vi "Running State Logic.vi"(8 "error in (no error)":errorcluster, 11 "CIFCorePlugin in":refnum<class "CIFCorePlugin.lvclass">) -> (0 "error out":errorcluster, 2 "Running State Logic":T1, 3 "CIFCorePlugin out":refnum<class "CIFCorePlugin.lvclass">)   [LabVIEW 2021, in "CIFCorePlugin.lvclass"]
uses:
  CIFCorePlugin.lvclass
  Typedef/Running State Logic.ctl
  CIFCorePlugin.lvclass/CIFCorePlugin.ctl
  Common/Typedef/Plugin State.ctl
  Common/CIFCoreCommon.lvlib
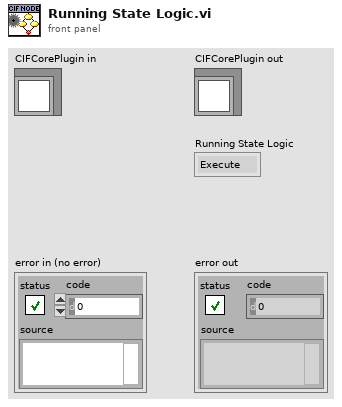
[diagram p1: front panel]
types:
  T1 = typedef "CIFCorePlugin.lvclass/Running State Logic.ctl" = enum16{"Execute", "Housekeep", "Cleanup", "Error", "Destroy"}
  T2 = typedef "CIFCorePlugin.lvclass/Energized States.ctl" = enum16{"Listen", "Prepare", "Execute", "Housekeep", "Cleanup", "Destroy"}
  T3 = typedef "CIFCoreCommon.lvlib/Plugin State.ctl" = enum32{"Null", "Creating", "Listening", "Running", "CleaningUp", "Destroying"}
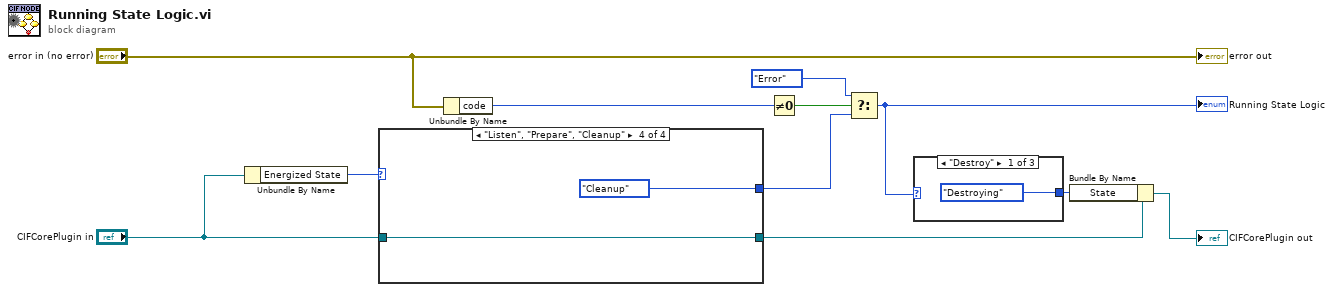
[diagram p0: block diagram]
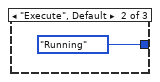
[diagram p2: hidden frame]
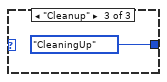
[diagram p3: hidden frame]
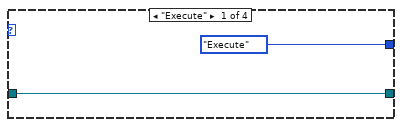
[diagram p4: hidden frame]
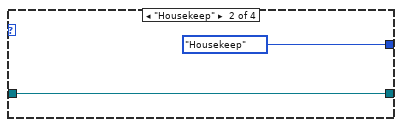
[diagram p5: hidden frame]
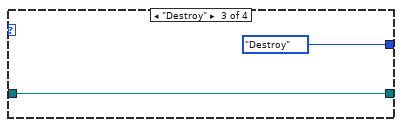
[diagram p6: hidden frame]
diagram:
  n1 = Unbundle By Name("CIFCorePlugin in") -> ("Energized State"=w8:T2)
  n2 = case shown="\"Listen\", \"Prepare\", \"Cleanup\"" w8 {
    tunnel: [Running_State_Logic."Execute" ("Execute State Logic") Running_State_Logic."Housekeep" ("Execute State Logic") Running_State_Logic."Destroy" ("Execute State Logic") Running_State_Logic."Cleanup" ("Execute State Logic")] -> w7
    tunnel: "CIFCorePlugin in" -> [w13 w15 w17 w19]
    tunnel: [w13 w15 w17 w19] -> w1
    frame "Execute" {
    }
    frame "Housekeep" {
    }
    frame "Destroy" {
    }
    frame "Listen", "Prepare", "Cleanup" {
    }
  }
  n3 = Unbundle By Name("error in (no error)") -> ("code"=w10:i32)
  n4 = Not Equal To 0?(x=w10) -> (x != 0?=w9:bool)
  n5 = Select(t=Running_State_Logic."Error" ("Execute State Logic"), s=w9, f=w7) -> (s? t:f=w4:T1)
  "Running State Logic" <- w4
  n6 = case shown="\"Destroy\"" w4 {
    tunnel: [Plugin_State."Destroying" ("Status.State") Plugin_State."Running" ("Status.State") Plugin_State."CleaningUp" ("Status.State")] -> w2
    frame "Destroy" {
    }
    frame "Execute", Default {
    }
    frame "Cleanup" {
    }
  }
  n7 = Bundle By Name(cluster=w1, "State"=w2) -> (→"CIFCorePlugin out":refnum<class "CIFCorePlugin.lvclass">)
  "error out" <- "error in (no error)"
